vi "25CA.vi"() -> ()   [LabVIEW 2017]
uses:
  <vilib>/Instr/_visa.llb/VISA Configure Serial Port (Instr).vi
panel:
  out "String 2":string
  out "Sensor 2":bool
  in  "COM PORT":refnum<visa-resource-name>
  out "Sensor 1":bool
  out "String":string
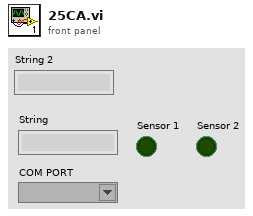
[diagram p1: front panel]
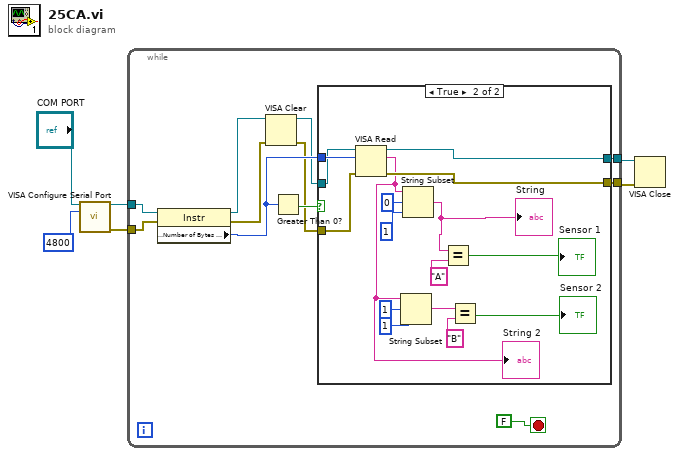
[diagram p0: block diagram]
diagram:
  n1 = call-poly "VISA Configure Serial Port"("VISA resource name"="COM PORT", "baud rate (9600)"=u32 4800) -> ("VISA resource name out"=w5:refnum<visa-resource-name>, "error out"=w4:errorcluster)  [unwired: 12 in]
  n2 = while {
    tunnel: w5 -> [w16]
    tunnel: w4 -> [w17]
    tunnel: [w14] -> w2
    tunnel: [w13] -> w1
    stop <- FALSE ("y") stop-if-true
    n3 = property class="Instr"(reference=w16, error in=w17) -> (reference out=w7:refnum<visa-resource-name>, error out=w8:errorcluster, "Serial Settings:Number of Bytes at Serial Port"=w15:u32)
    n4 = VISA Clear(VISA resource name=w7, error in (no error)=w8) -> (VISA resource name out=w10:refnum<visa-resource-name>, error out=w9:errorcluster)
    n5 = Greater Than 0?(x=w15) -> (x > 0?=w12:bool)
    n6 = case shown="True" w12 {
      tunnel: w9 -> [w19 w32]
      tunnel: w15 -> [_ w34]
      tunnel: w10 -> [w18 w33]
      tunnel: [w18 w31] -> w14
      tunnel: [w19 w30] -> w13
      frame False {
      }
      frame True {
        n7 = VISA Read(VISA resource name=w33, byte count=w34, error in (no error)=w32) -> (VISA resource name out=w31:refnum<visa-resource-name>, read buffer=w22:string, error out=w30:errorcluster)  [unwired: 1 out]
        "String 2" <- w22
        n8 = String Subset(string=w22, offset (0)=1, length (rest)=1 ("length (rest)")) -> (substring=w26:string)
        n9 = String Subset(string=w22, offset (0)=0, length (rest)=1 ("length (rest)")) -> (substring=w23:string)
        "String" <- w23
        n10 = Equal?(x=w23, y="A") -> (x = y?=→"Sensor 1":bool)
        n11 = Equal?(x=w26, y="B") -> (x = y?=→"Sensor 2":bool)
      }
    }
  }
  n12 = VISA Close(VISA resource name=w2, error in (no error)=w1) -> ()  [unwired: 1 out]
